vi "Init.vi"(10 "Players number in":i32=4) -> (3 "Communication out":refnum<class "Communication.lvclass">, 5 "Stop User Event out":refnum<user-event>)   [LabVIEW 2021, in "Communication.lvclass"]
doc: "MIT Licence\nCopyright (c) 2024 David Grollier"
uses:
  Communication.lvclass
  Game Componants/Game Board/State Command.ctl
  Game Componants/Game Board/Action Command.ctl
  Communication.lvclass/Communication.ctl
  Game Componants/Game Board/Game Board.lvclass
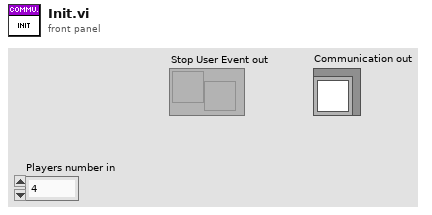
[diagram p1: front panel]
types:
  T1 = typedef "Game Board.lvclass/Action Command.ctl" = cluster{"Boost":bool}
  T2 = typedef "Game Board.lvclass/State Command.ctl" = cluster{"Direction":cluster{dbl, dbl}, "Velocity":dbl}
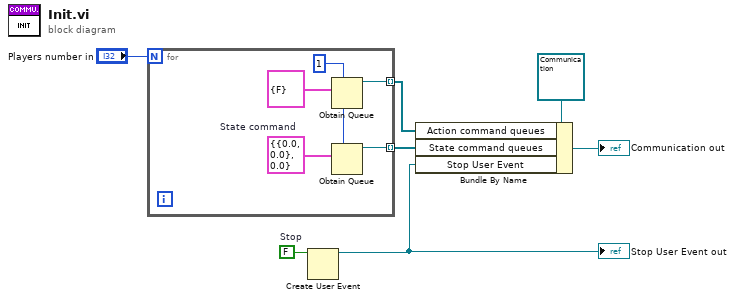
[diagram p0: block diagram]
diagram:
  w2 = FALSE  # Stop
  n1 = for {
    N: "Players number in" -> [_]
    tunnel: [w11] -> w4 mode=indexing
    tunnel: [w9] -> w3 mode=indexing
    w8 = 1 ("max queue size (-1, unlimited)")
    w10 = T2 {"Direction"={0.0, 0.0}, "Velocity"=0.0}  # State command
    n2 = Obtain Queue(max queue size (-1, unlimited)=w8, element data type=T1 {"Boost"=FALSE} ("Action commands")) -> (queue out=w11:refnum<queue>)  [unwired: 3 in, 2 out]
    n3 = Obtain Queue(max queue size (-1, unlimited)=w8, element data type=w10) -> (queue out=w9:refnum<queue>)  [unwired: 3 in, 2 out]
  }
  n4 = Create User Event(user event datatype=w2) -> (user event=w1:refnum<user-event>)  [unwired: 1 in, 1 out]
  "Stop User Event out" <- w1
  n5 = Bundle By Name(cluster=refnum<class "Communication.lvclass"> refnum ("Communication out"), "Action command queues"=w4, "State command queues"=w3, "Stop User Event"=w1) -> (→"Communication out":refnum<class "Communication.lvclass">)
